vi "Read Data Preview.vi"(8 "error in (no error)":errorcluster, 11 "Data Value Reference in":refnum<data-value>) -> (0 "error out":errorcluster, 2 "Data":u64[](array[numeric]), 3 "Data Value Reference out":refnum<data-value>)   [LabVIEW 2016]
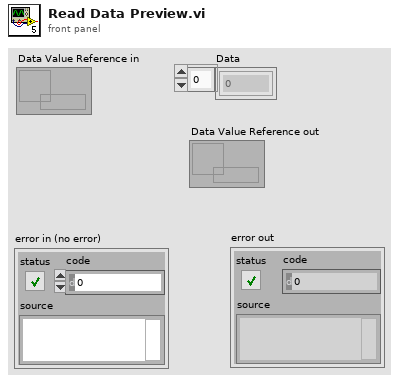
[diagram p1: front panel]
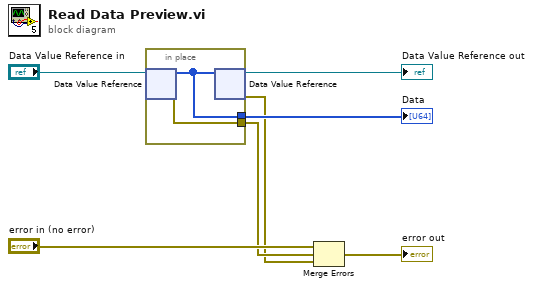
[diagram p0: block diagram]
diagram:
  n1 = in-place {
    in-place-border: [w9] -> w7
    in-place-border: [w8] -> w3
    n2 = in-place-dvr #1("Data Value Reference in") -> (w9:u64[], w8:errorcluster)
    n3 = in-place-dvr #1(w9) -> (→"Data Value Reference out":refnum<data-value>, w2:errorcluster)
  }
  "Data" <- w7
  n4 = Merge Errors("error in (no error)", w3, w2) -> (→"error out":errorcluster)
